vi "Read Data.vi"(8 "error in (no error)":errorcluster, 11 "HP53181 in":refnum<class "HP53181.lvclass">) -> (0 "error out":errorcluster, 2 "Data":waveform(dbl)[](array[waveform]), 3 "HP53181 out":refnum<class "HP53181.lvclass">)   [LabVIEW 2015, in "HP53181.lvclass"]
uses:
  HP53181.lvclass
  Instrument/Instrument.lvclass
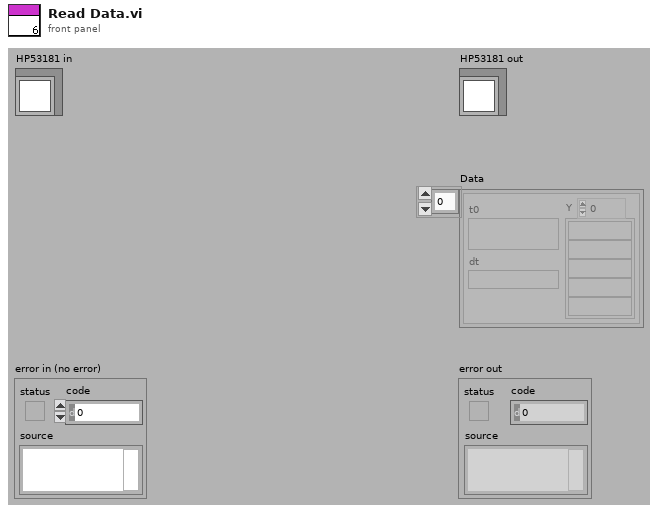
[diagram p1: front panel]
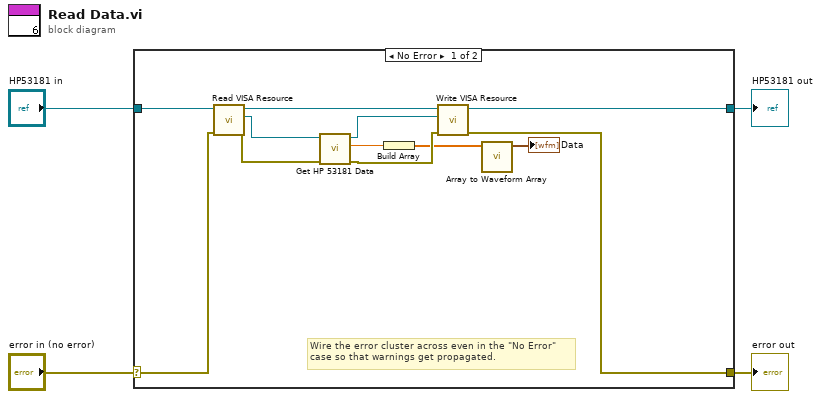
[diagram p0: block diagram]
diagram:
  n1 = case shown="No Error" "error in (no error)" {
    selector: "error in (no error)" -> [w11 w18]
    tunnel: [w7 w18] -> w3
    tunnel: [w14 w17] -> w1
    tunnel: "HP53181 in" -> [w16 w17]
    frame No Error {
      # "Wire the error cluster across even in the \"No Error\"\ncase so that warnings get propagated."
      n2 = call "Read VISA Resource.vi"("error in (no error)"=w11, "Instrument.lvclass in"=w16) -> ("error out"=w10:errorcluster, "VISA Resource"=w13:refnum<visa-resource-name>, "Instrument.lvclass out"=w15:refnum<class "HP53181.lvclass">)  [unwired: 7 out]
      n3 = call "Get HP 53181 Data.vi"("error in (no error)"=w10, "VISA Resource Name"=w13) -> ("error out"=w8:errorcluster, "Data"=w9:dbl, "VISA Resource Name Out"=w12:refnum<visa-resource-name>)  [unwired: 6 out]
      n4 = Build Array(w9) -> (w5:dbl[])
      n5 = call "Write VISA Resource.vi"("error in (no error)"=w8, "VISA Resource"=w12, "Instrument.lvclass in"=w15) -> ("error out"=w7:errorcluster, "Instrument.lvclass out"=w14:refnum<class "HP53181.lvclass">)  [unwired: 7 out]
      n6 = call "Array to Waveform Array.vi"("Array"=w5) -> ("Waveform"=→"Data":waveform(dbl)[])  [unwired: 10 in]
    }
    frame Error {
    }
  }
  "error out" <- w3
  "HP53181 out" <- w1
